vi "Write TIFF.vi"(8 "error in (no error)":errorcluster, 10 "Path":path, 11 "ImageHandler in":refnum<class "ImageHandler.lvclass">) -> (0 "error out":errorcluster, 3 "ImageHandler out":refnum<class "ImageHandler.lvclass">)   [LabVIEW 2022 SP3, in "ImageHandler.lvlib" / "ImageHandler.lvclass"]
uses:
  ImageHandler.lvclass
  ImageHandler.lvclass/ImageHandler.ctl
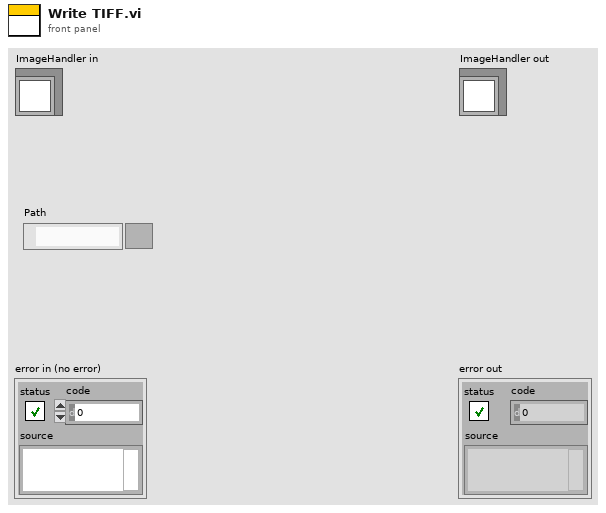
[diagram p1: front panel]
types:
  T1 = typedef "IMAQ Image.ctl" = refnum<image>
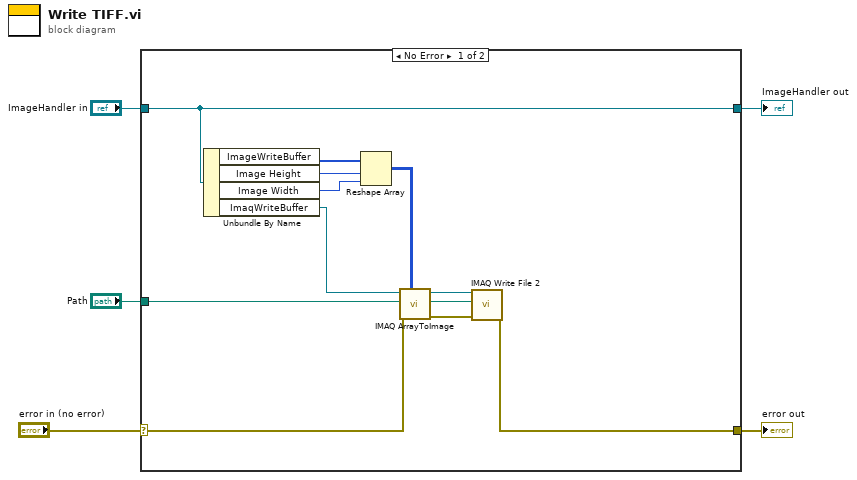
[diagram p0: block diagram]
diagram:
  n1 = case shown="No Error" "error in (no error)" {
    selector: "error in (no error)" -> [w15 w18]
    tunnel: [w14 w18] -> w4
    tunnel: [w16 w17] -> w2
    tunnel: "ImageHandler in" -> [w16 w17]
    tunnel: "Path" -> [w13 _]
    frame No Error {
      n2 = Unbundle By Name(w16) -> ("ImageWriteBuffer"=w9:u16[], "Image Height"=w10:i32, "Image Width"=w11:i32, "ImaqWriteBuffer"=w7:T1)
      n3 = Reshape Array(w9, w10, w11) -> (w8:u16[][])
      n4 = call "IMAQ ArrayToImage"("Image Pixels (U16)"=w8, "error in (no error)"=w15, "Image"=w7) -> ("error out"=w12:errorcluster, "Image Out"=w6:T1)  [unwired: 7 in]
      n5 = call-poly "IMAQ Write File 2"("error in (no error)"=w12, "File Path"=w13, "Image"=w6) -> ("error out"=w14:errorcluster)  [unwired: 7 in, 1 out]
    }
    frame Error {
    }
  }
  "error out" <- w4
  "ImageHandler out" <- w2
